vi "InitializeFpga.vi"(8 "error in":errorcluster) -> (0 "error out":errorcluster)   [LabVIEW 2015]
uses:
  <vilib>/rvi/interface/RandomDataEmulation/nirviRandomDataOpen.vi
  <vilib>/rvi/errors/niLvFpgaMergeErrorWithErrorCode.vi
  <vilib>/rvi/interface/RandomDataEmulation/nirviRandomDataRunMethod.vi
  <vilib>/rvi/interface/RandomDataEmulation/nirviRandomDataDMAMethods.vi
  GlobalVariables.vi
  <vilib>/rvi/interface/nirviOpenFPGA/nirviOpenFPGA.xnode
  Fpga-Version/PXI-7953R/Fft.vi
  <vilib>/rvi/interface/nirviMethod/nirviMethod.xnode
  <vilib>/FPGA/interface/niFpgaViExecutionMode.ctl
panel:
  out "FPGA VI Reference Out":refnum<k20>
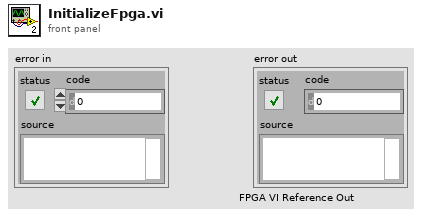
[diagram p1: front panel]
types:
  T1 = typedef "niFpgaViExecutionMode.ctl" = enum16{"FPGA Target", "Simulation (Simulated I/O)", "Simulation (Real I/O)", "Third-Party Simulation"}
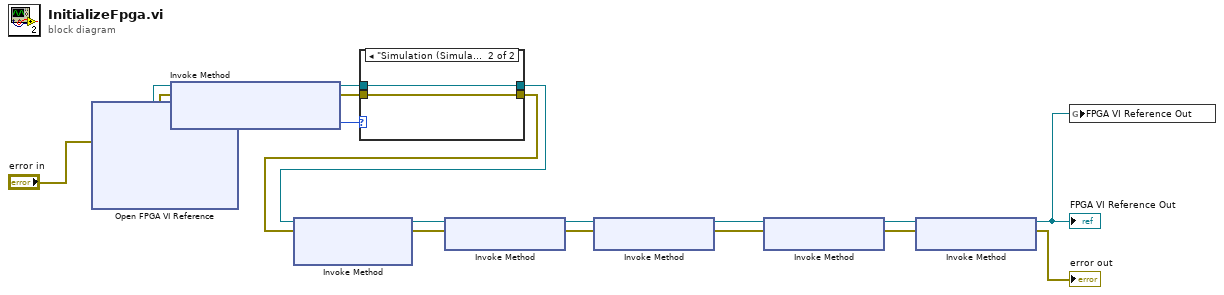
[diagram p0: block diagram]
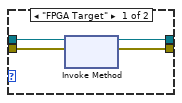
[diagram p2: hidden frame]
diagram:
  n1 = xnode "Open FPGA VI Reference"("error in"="error in") -> ("FPGA VI Reference Out"=w15:refnum<k20>, "error out"=w10:errorcluster)  [unwired: 1 in]
  n2 = xnode "Invoke Method"("FPGA VI Reference In"=w15, "error in"=w10) -> ("FPGA VI Reference Out"=w13:refnum<k20>, "error out"=w12:errorcluster, "FPGA VI Execution Mode"=w14:T1)
  n3 = case shown="\"Simulation (Simulated I/O)\", Default" w14 {
    tunnel: [w22 w23] -> w7
    tunnel: [w21 w24] -> w11
    tunnel: w13 -> [w20 w24]
    tunnel: w12 -> [w19 w23]
    frame "FPGA Target" {
      n4 = xnode "Invoke Method"("FPGA VI Reference In"=w20, "error in"=w19) -> ("FPGA VI Reference Out"=w21:refnum<k20>, "error out"=w22:errorcluster)
    }
    frame "Simulation (Simulated I/O)", Default {
    }
  }
  n5 = xnode "Invoke Method"("FPGA VI Reference In"=w11, "error in"=w7) -> ("FPGA VI Reference Out"=w8:refnum<k20>, "error out"=w1:errorcluster)  [unwired: 1 in]
  n6 = xnode "Invoke Method"("FPGA VI Reference In"=w8, "error in"=w1) -> ("FPGA VI Reference Out"=w5:refnum<k20>, "error out"=w2:errorcluster)
  n7 = xnode "Invoke Method"("FPGA VI Reference In"=w5, "error in"=w2) -> ("FPGA VI Reference Out"=w4:refnum<k20>, "error out"=w3:errorcluster)
  n8 = xnode "Invoke Method"("FPGA VI Reference In"=w4, "error in"=w3) -> ("FPGA VI Reference Out"=w17:refnum<k20>, "error out"=w18:errorcluster)
  n9 = xnode "Invoke Method"("FPGA VI Reference In"=w17, "error in"=w18) -> ("FPGA VI Reference Out"=w6:refnum<k20>, "error out"=→"error out":errorcluster)
  "FPGA VI Reference Out" <- w6
  n10 = global write "GlobalVariables.vi" "FPGA VI Reference Out"(w6) -> ()
